vi "Get All Folders.vi"() -> ()   [LabVIEW 2020]
panel:
  out "Array 2":path[](array[path])
  out "Array":path[](array[path])
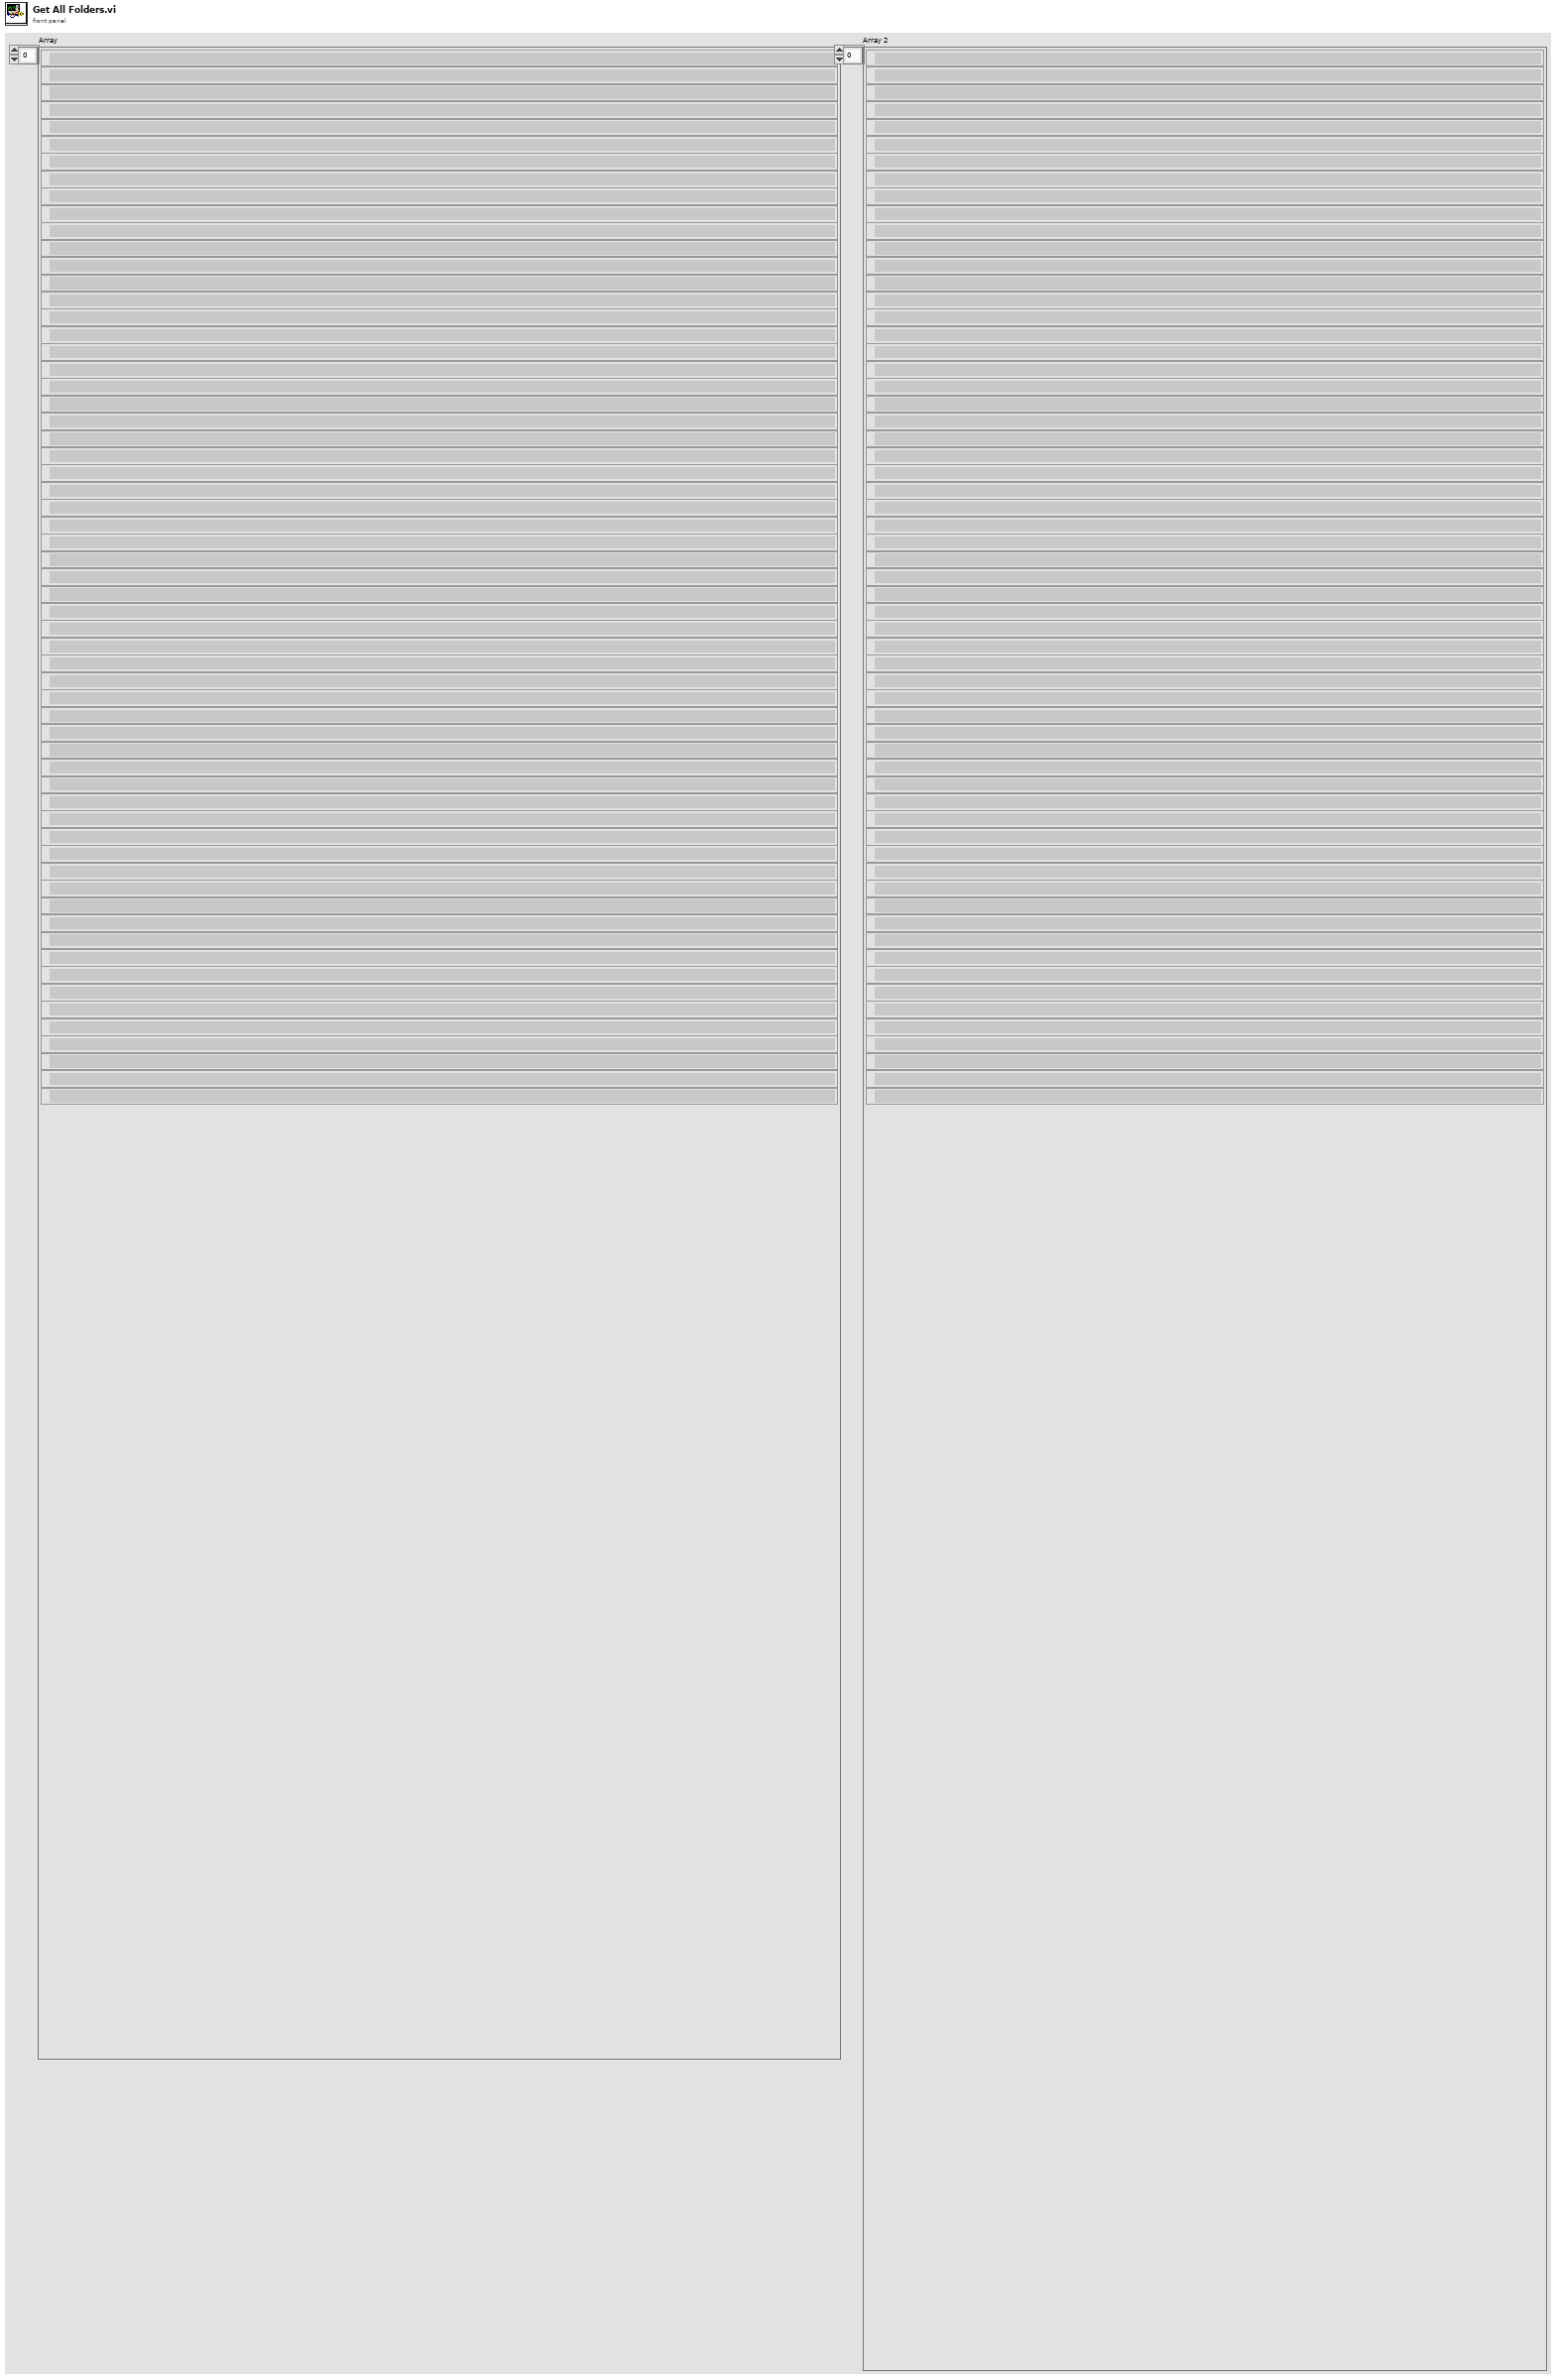
[diagram p1: front panel]
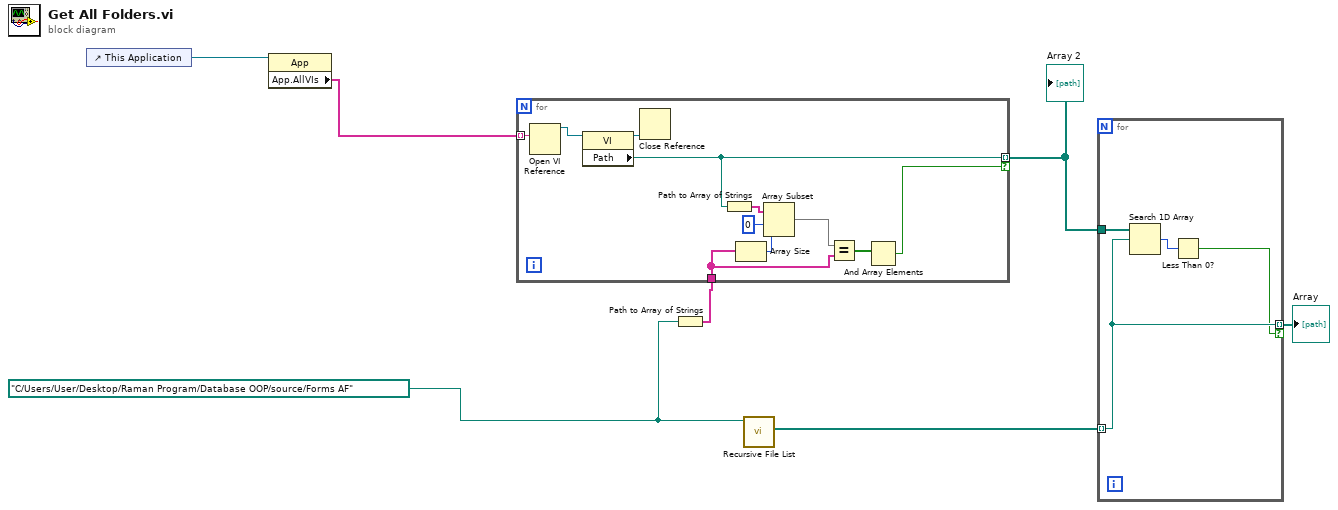
[diagram p0: block diagram]
diagram:
  w2 = path "C:/Users/User/Desktop/Raman Program/Database OOP/source/Forms AF"
  n1 = control-ref of="This Application"() -> (w7:refnum<vi>)
  n2 = property class="App"(reference=w7) -> ("App.AllVIs"=w6:string[])  [unwired: 1 in, 2 out]
  n3 = Path to Array of Strings(0:w2) -> (2:w1:string[])  [unwired: 1 out]
  n4 = for {
    tunnel: w6 -> [w18] mode=indexing
    tunnel: [w15] -> w4 mode=indexing if=w8
    tunnel: w1 -> [w11]
    n5 = Open VI Reference(vi path=w18) -> (vi reference=w17:refnum<vi>)  [unwired: 5 in, 1 out]
    n6 = property class="VI"(reference=w17) -> (reference out=w16:refnum<vi>, "Path"=w15:path)  [unwired: 1 in, 1 out]
    n7 = Close Reference(reference=w16) -> ()  [unwired: 1 in, 1 out]
    n8 = Path to Array of Strings(0:w15) -> (2:w14:string[])  [unwired: 1 out]
    n9 = Array Size(array=w11) -> (size(s)=w12:i32)
    n10 = Array Subset(array=w14, index=0, length=w12) -> (w10:string[])
    n11 = Equal?(x=w10, y=w11) -> (x = y?=w9:bool[])
    n12 = And Array Elements(Boolean array=w9) -> (logical AND=w8:bool)
  }
  "Array 2" <- w4
  n13 = call <vilib>:"Recursive File List.vi"("Folder Path"=w2) -> ("All Files in Dir"=w5:path[])  [unwired: 6 in, 4 out]
  n14 = for {
    tunnel: w5 -> [w21] mode=indexing
    tunnel: w4 -> [w22]
    tunnel: [w21] -> w3 mode=indexing if=w19
    n15 = Search 1D Array(1D array=w22, element=w21) -> (index of element=w20:i32)  [unwired: 1 in]
    n16 = Less Than 0?(x=w20) -> (x < 0?=w19:bool)
  }
  "Array" <- w3
